vi "Autonics_XYScan.vi"() -> ()   [LabVIEW 2018]
uses:
  <vilib>/Instr/_visa.llb/VISA Configure Serial Port (Instr).vi
panel:
  in  "FB Move Distance (mm)":dbl=1.0
  out "FB Current  Position (mm)":dbl format="%#_4g"
  in  "COM FB":refnum<visa-resource-name>="COM3"
  in  "Backward":bool
  in  "Forward":bool
  in  "Multiplier":dbl=10.0
  in  "Travel per Pulse (mm)":dbl=0.004
  out "LR Current  Position (mm)":dbl format="%#_4g"
  in  "Flow control":u16(ring) items=["None", "XON/XOFF", "RTS/CTS", "XON/XOFF & RTS/CTS", "DTR/DSR", "XON/XOFF & DTR/DSR"]
  in  "Stop bits":u16(ring)=10 items=["1.0"=10, "1.5"=15, "2.0"=20]
  in  "Speed (mm/s)":dbl=0.5
  in  "LR Move Distance (mm)":dbl=1.0
  in  "Stop":bool
  in  "Home":bool
  in  "Left":bool
  in  "Right":bool
  in  "Stop Scan":bool
  in  "Parity":dbl
  in  "Data bits":u16=8 min=5 max=8 step=1
  in  "Baud Rate":u32=9600
  in  "COM LR":refnum<visa-resource-name>="COM3"
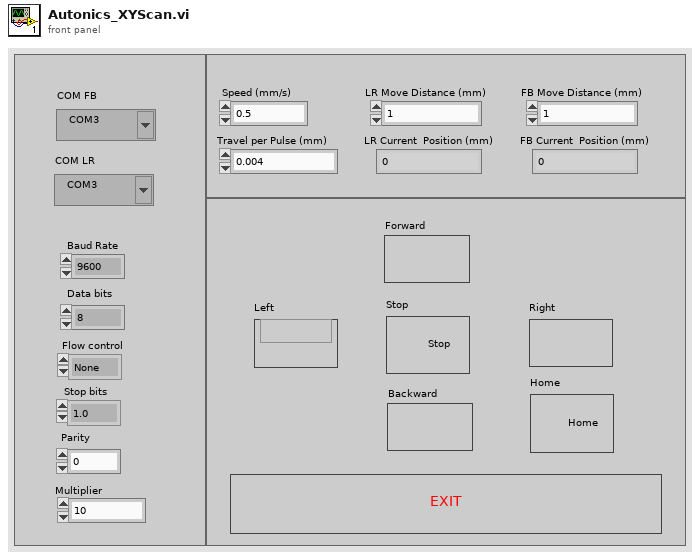
[diagram p1: front panel]
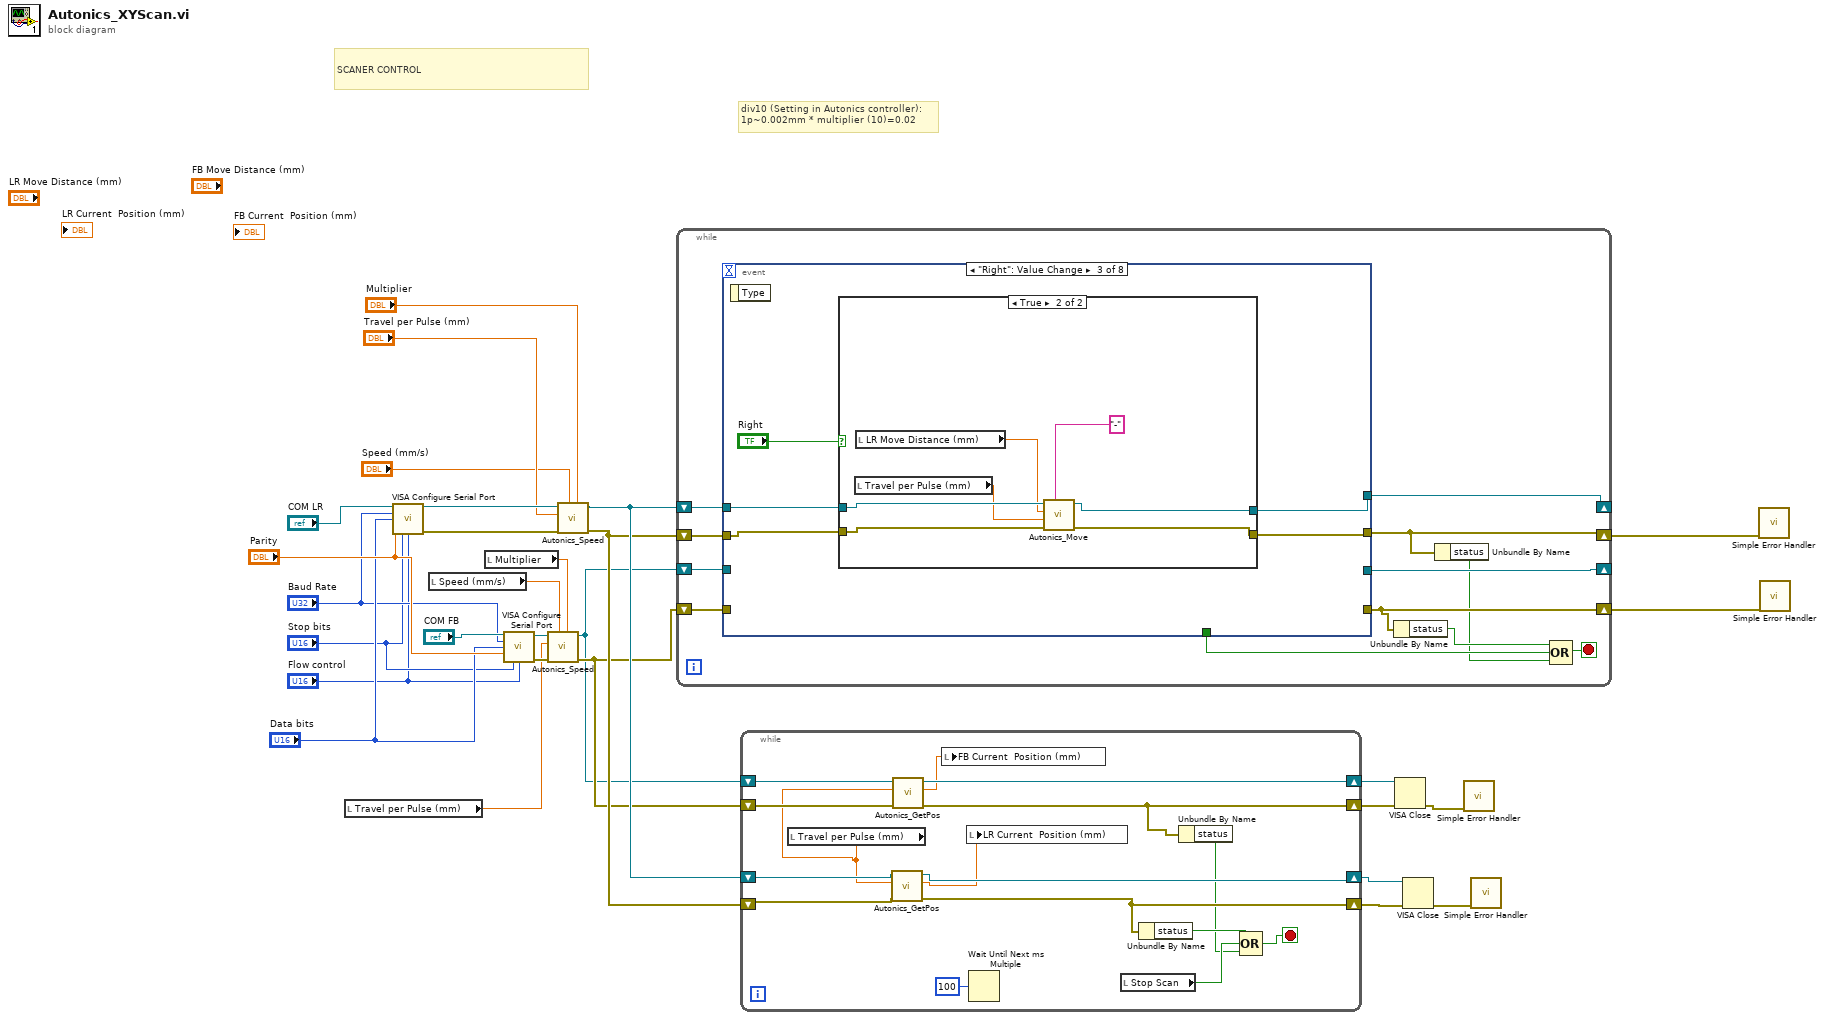
[diagram p0: block diagram]
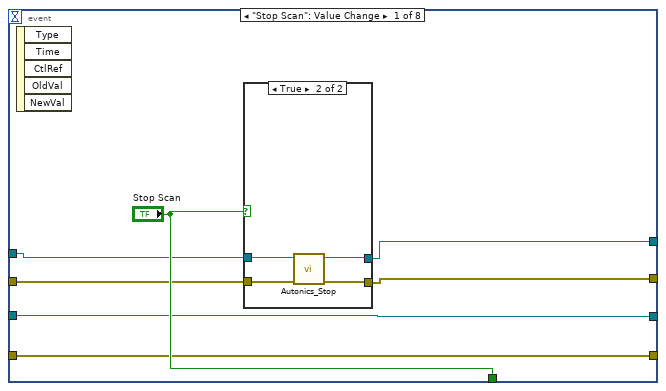
[diagram p2: hidden frame]
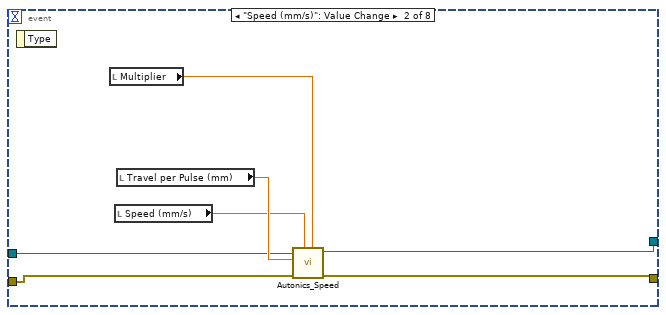
[diagram p4: hidden frame]
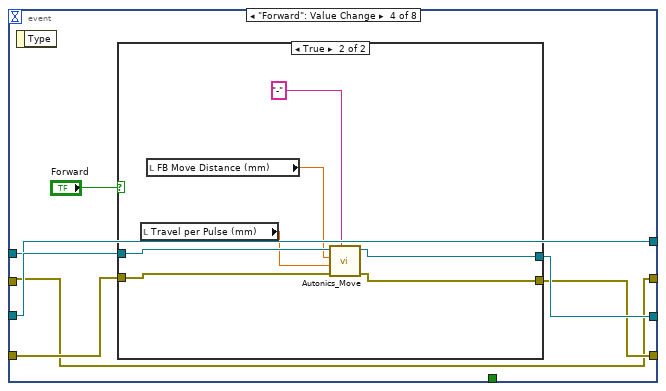
[diagram p6: hidden frame]
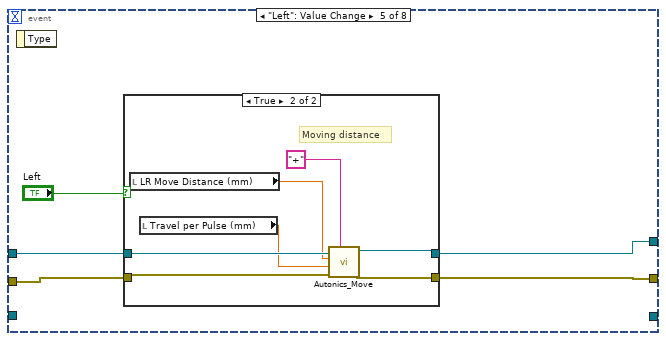
[diagram p8: hidden frame]
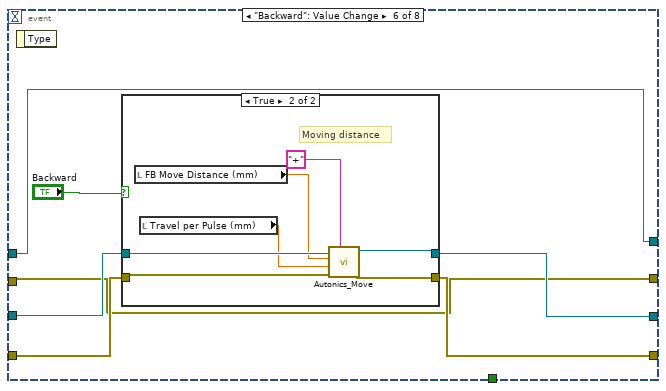
[diagram p10: hidden frame]
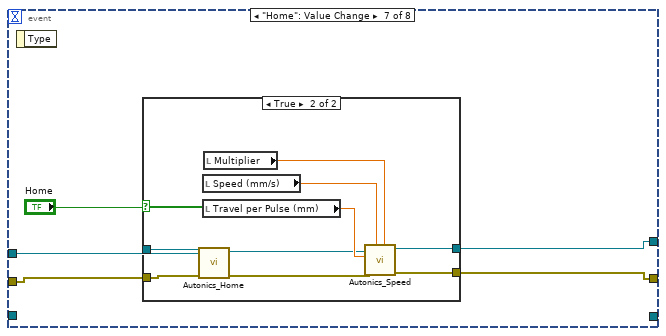
[diagram p12: hidden frame]
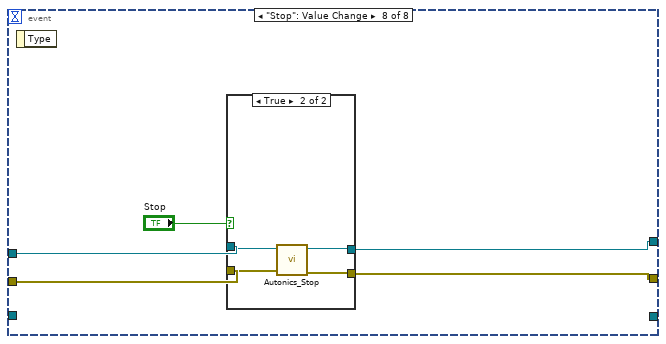
[diagram p14: hidden frame]
diagram:
  # "div10 (Setting in Autonics controller):\n1p~0.002mm * multiplier (10)=0.02"
  # "SCANER CONTROL"
  n1 = local read "Travel per Pulse (mm)"() -> (w11:dbl)
  n2 = call-poly "VISA Configure Serial Port"("VISA resource name"="COM LR", "baud rate (9600)"="Baud Rate", "data bits (8)"="Data bits", "parity (0:none)"="Parity", "stop bits (10: 1 bit)"="Stop bits", "flow control (0:none)"="Flow control") -> ("VISA resource name out"=w22:refnum<visa-resource-name>, "error out"=w21:errorcluster)  [unwired: 8 in]
  n3 = local read "Speed (mm/s)"() -> (w13:dbl)
  n4 = local read "Multiplier"() -> (w12:dbl)
  n5 = call-poly "VISA Configure Serial Port"("VISA resource name"="COM FB", "baud rate (9600)"="Baud Rate", "data bits (8)"="Data bits", "parity (0:none)"="Parity", "stop bits (10: 1 bit)"="Stop bits", "flow control (0:none)"="Flow control") -> ("VISA resource name out"=w17:refnum<visa-resource-name>, "error out"=w16:errorcluster)  [unwired: 8 in]
  n6 = call "Autonics_Speed.vi"("Multiplier"=w12, "Speed (mm/s)"=w13, "error in (no error)"=w16, "Travel per  Pulse"=w11, "VISA resource name"=w17) -> ("error out"=w5:errorcluster, "VISA resource name out"=w4:refnum<visa-resource-name>)  [unwired: 5 in]
  n7 = call "Autonics_Speed.vi"("Multiplier"="Multiplier", "Speed (mm/s)"="Speed (mm/s)", "error in (no error)"=w21, "Travel per  Pulse"="Travel per Pulse (mm)", "VISA resource name"=w22) -> ("error out"=w23:errorcluster, "VISA resource name out"=w24:refnum<visa-resource-name>)  [unwired: 5 in]
  n8 = while {
    shift-right: [w41] -> _
    shift-left: w24 -> [w40]
    shift-right: [w31] -> w27
    shift-left: w23 -> [w39]
    shift-right: [w34] -> _
    shift-left: w4 -> [w36]
    shift-right: [w33] -> w15
    shift-left: w5 -> [w35]
    stop <- w38 stop-if-true
    n9 = event shown="[2] \"Right\": Value Change" {
      selector: _ -> [_ _ _ _ _ _ _ _]
      dyn-events: _ -> [_ _ _ _ _ _ _ _]
      timeout: _ -> [_ _ _ _ _ _ _ _]
      tunnel: w40 -> [w47 w60 w64 w77 w94 w107 w126 w140]
      tunnel: w39 -> [w46 w59 w63 w76 w93 w106 w125 w139]
      tunnel: [w45 w58 w66 w77 w96 w107 w123 w142] -> w41
      tunnel: [w44 w57 w65 w76 w95 w106 w122 w141] -> w31
      tunnel: ["Stop Scan" _ _ _ _ _ _ _] -> w37
      tunnel: w36 -> [w42 _ _ w81 _ w110 _ _]
      tunnel: w35 -> [w43 _ _ w80 _ w111 _ _]
      tunnel: [w42 _ _ w79 _ w108 _ _] -> w34
      tunnel: [w43 _ _ w78 _ w109 _ _] -> w33
      event "Stop Scan": Value Change {
        n10 = event-data() -> ()  [unwired: 1 in, 5 out]
        n11 = case shown="True" "Stop Scan" {
          tunnel: [w50 w53] -> w45
          tunnel: [w49 w54] -> w44
          tunnel: w47 -> [w50 w52]
          tunnel: w46 -> [w49 w51]
          frame False {
          }
          frame True {
            n12 = call "Autonics_Stop.vi"("error in (no error)"=w51, "VISA resource name"=w52) -> ("error out"=w54:errorcluster, "VISA resource name out"=w53:refnum<visa-resource-name>)  [unwired: 8 in]
          }
        }
      }
      event "Speed (mm/s)": Value Change {
        n13 = event-data() -> ()  [unwired: 1 in, 1 out]
        n14 = local read "Multiplier"() -> (w55:dbl)
        n15 = local read "Speed (mm/s)"() -> (w56:dbl)
        n16 = local read "Travel per Pulse (mm)"() -> (w61:dbl)
        n17 = call "Autonics_Speed.vi"("Multiplier"=w55, "Speed (mm/s)"=w56, "error in (no error)"=w59, "Travel per  Pulse"=w61, "VISA resource name"=w60) -> ("error out"=w57:errorcluster, "VISA resource name out"=w58:refnum<visa-resource-name>)  [unwired: 5 in]
      }
      event "Right": Value Change {
        n18 = event-data() -> ()  [unwired: 1 in, 1 out]
        n19 = case shown="True" "Right" {
          tunnel: [w67 w73] -> w66
          tunnel: [w68 w69] -> w65
          tunnel: w64 -> [w67 w75]
          tunnel: w63 -> [w68 w74]
          frame False {
          }
          frame True {
            n20 = local read "Travel per Pulse (mm)"() -> (w71:dbl)
            n21 = local read "LR Move Distance (mm)"() -> (w72:dbl)
            n22 = call "Autonics_Move.vi"("Direction (+)"="-", "error in (no error)"=w74, "Travel per Pulse (mm)"=w71, "Move Distance (mm)"=w72, "VISA resource name"=w75) -> ("error out"=w69:errorcluster, "VISA resource name out"=w73:refnum<visa-resource-name>)  [unwired: 5 in]
          }
        }
      }
      event "Forward": Value Change {
        n23 = event-data() -> ()  [unwired: 1 in, 1 out]
        n24 = case shown="True" "Forward" {
          tunnel: [w83 w89] -> w79
          tunnel: [w84 w88] -> w78
          tunnel: w81 -> [w83 w91]
          tunnel: w80 -> [w84 w90]
          frame False {
          }
          frame True {
            n25 = local read "Travel per Pulse (mm)"() -> (w86:dbl)
            n26 = local read "FB Move Distance (mm)"() -> (w87:dbl)
            n27 = call "Autonics_Move.vi"("Direction (+)"="-", "error in (no error)"=w90, "Travel per Pulse (mm)"=w86, "Move Distance (mm)"=w87, "VISA resource name"=w91) -> ("error out"=w88:errorcluster, "VISA resource name out"=w89:refnum<visa-resource-name>)  [unwired: 5 in]
          }
        }
      }
      event "Left": Value Change {
        n28 = event-data() -> ()  [unwired: 1 in, 1 out]
        n29 = case shown="True" "Left" {
          tunnel: [w98 w103] -> w96
          tunnel: [w97 w102] -> w95
          tunnel: w94 -> [w98 w105]
          tunnel: w93 -> [w97 w104]
          frame False {
          }
          frame True {
            # "Moving distance"
            n30 = local read "LR Move Distance (mm)"() -> (w100:dbl)
            n31 = local read "Travel per Pulse (mm)"() -> (w99:dbl)
            n32 = call "Autonics_Move.vi"("Direction (+)"="+", "error in (no error)"=w104, "Travel per Pulse (mm)"=w99, "Move Distance (mm)"=w100, "VISA resource name"=w105) -> ("error out"=w102:errorcluster, "VISA resource name out"=w103:refnum<visa-resource-name>)  [unwired: 5 in]
          }
        }
      }
      event "Backward": Value Change {
        n33 = event-data() -> ()  [unwired: 1 in, 1 out]
        n34 = case shown="True" "Backward" {
          tunnel: [w114 w119] -> w108
          tunnel: [w113 w118] -> w109
          tunnel: w110 -> [w114 w121]
          tunnel: w111 -> [w113 w120]
          frame False {
          }
          frame True {
            # "Moving distance"
            n35 = local read "FB Move Distance (mm)"() -> (w116:dbl)
            n36 = local read "Travel per Pulse (mm)"() -> (w115:dbl)
            n37 = call "Autonics_Move.vi"("Direction (+)"="+", "error in (no error)"=w120, "Travel per Pulse (mm)"=w115, "Move Distance (mm)"=w116, "VISA resource name"=w121) -> ("error out"=w118:errorcluster, "VISA resource name out"=w119:refnum<visa-resource-name>)  [unwired: 5 in]
          }
        }
      }
      event "Home": Value Change {
        n38 = event-data() -> ()  [unwired: 1 in, 1 out]
        n39 = case shown="True" "Home" {
          tunnel: [w128 w130] -> w123
          tunnel: [w127 w129] -> w122
          tunnel: w126 -> [w128 w137]
          tunnel: w125 -> [w127 w136]
          frame False {
          }
          frame True {
            n40 = call "Autonics_Home.vi"("error in (no error)"=w136, "VISA resource name"=w137) -> ("error out"=w131:errorcluster, "VISA resource name out"=w132:refnum<visa-resource-name>)  [unwired: 8 in]
            n41 = local read "Speed (mm/s)"() -> (w134:dbl)
            n42 = local read "Travel per Pulse (mm)"() -> (w135:dbl)
            n43 = local read "Multiplier"() -> (w133:dbl)
            n44 = call "Autonics_Speed.vi"("Multiplier"=w133, "Speed (mm/s)"=w134, "error in (no error)"=w131, "Travel per  Pulse"=w135, "VISA resource name"=w132) -> ("error out"=w129:errorcluster, "VISA resource name out"=w130:refnum<visa-resource-name>)  [unwired: 5 in]
          }
        }
      }
      event "Stop": Value Change {
        n45 = event-data() -> ()  [unwired: 1 in, 1 out]
        n46 = case shown="True" "Stop" {
          tunnel: [w144 w145] -> w142
          tunnel: [w143 w148] -> w141
          tunnel: w140 -> [w144 w147]
          tunnel: w139 -> [w143 w146]
          frame False {
          }
          frame True {
            n47 = call "Autonics_Stop.vi"("error in (no error)"=w146, "VISA resource name"=w147) -> ("error out"=w148:errorcluster, "VISA resource name out"=w145:refnum<visa-resource-name>)  [unwired: 8 in]
          }
        }
      }
    }
    n48 = Unbundle By Name(w33) -> ("status"=w32:bool)
    n49 = Unbundle By Name(w31) -> ("status"=w30:bool)
    n50 = Compound Arithmetic op=OR(w32, w37, w30) -> (w38:bool)
  }
  n51 = while {
    shift-right: [w158] -> w26
    shift-left: w24 -> [w160]
    shift-right: [w157] -> w25
    shift-left: w23 -> [w159]
    shift-right: [w153] -> w3
    shift-left: w4 -> [w154]
    shift-right: [w152] -> w2
    shift-left: w5 -> [w155]
    stop <- w161 stop-if-true
    n52 = local read "Travel per Pulse (mm)"() -> (w149:dbl)
    n53 = call "Autonics_GetPos.vi"("error in (no error)"=w159, "Travel per Pulse (mm)"=w149, "VISA resource name"=w160) -> ("error out"=w157:errorcluster, "Current  Position (mm)"=w156:dbl, "VISA resource name out"=w158:refnum<visa-resource-name>)  [unwired: 6 in]
    n54 = call "Autonics_GetPos.vi"("error in (no error)"=w155, "Travel per Pulse (mm)"=w149, "VISA resource name"=w154) -> ("error out"=w152:errorcluster, "Current  Position (mm)"=w150:dbl, "VISA resource name out"=w153:refnum<visa-resource-name>)  [unwired: 6 in]
    n55 = local write "FB Current  Position (mm)"(w150) -> ()
    n56 = local write "LR Current  Position (mm)"(w156) -> ()
    n57 = Wait Until Next ms Multiple(millisecond multiple=u32 100) -> ()  [unwired: 1 out]
    n58 = local read "Stop Scan"() -> (w162:bool)
    n59 = Unbundle By Name(w157) -> ("status"=w163:bool)
    n60 = Unbundle By Name(w152) -> ("status"=w151:bool)
    n61 = Compound Arithmetic op=OR(w163, w162, w151) -> (w161:bool)
  }
  n62 = VISA Close(VISA resource name=w3, error in (no error)=w2) -> (error out=w1:errorcluster)
  n63 = VISA Close(VISA resource name=w26, error in (no error)=w25) -> (error out=w28:errorcluster)
  n64 = call <vilib>:"Simple Error Handler.vi"("error in (no error)"=w1) -> ()  [unwired: 4 in, 5 out]
  n65 = call <vilib>:"Simple Error Handler.vi"("error in (no error)"=w28) -> ()  [unwired: 4 in, 5 out]
  n66 = call <vilib>:"Simple Error Handler.vi"("error in (no error)"=w27) -> ()  [unwired: 4 in, 5 out]
  n67 = call <vilib>:"Simple Error Handler.vi"("error in (no error)"=w15) -> ()  [unwired: 4 in, 5 out]
